vi "Write passerId.vi"(8 "error in (no error)":errorcluster, 10 "passerId":u8, 11 "PositionTactic in":refnum<class "PositionTactic.lvclass">) -> (0 "error out":errorcluster, 3 "PositionTactic out":refnum<class "PositionTactic.lvclass">)   [LabVIEW 2023, in "PositionTactic.lvclass"]
uses:
  PositionTactic.lvclass
  PositionTactic.lvclass/PositionTactic.ctl
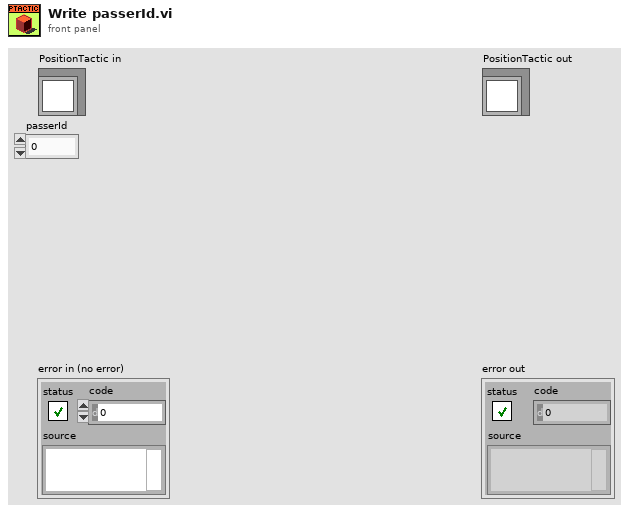
[diagram p1: front panel]
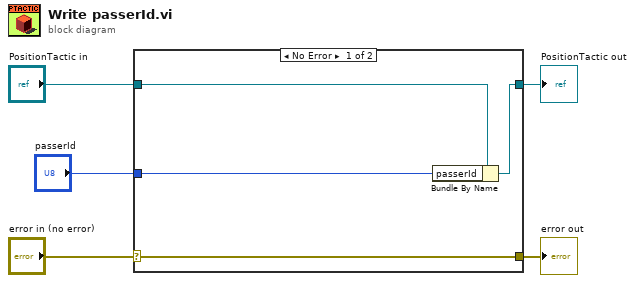
[diagram p0: block diagram]
diagram:
  n1 = case shown="No Error" "error in (no error)" {
    selector: "error in (no error)" -> [w9 w10]
    tunnel: [w9 w10] -> w4
    tunnel: [w7 w11] -> w2
    tunnel: "PositionTactic in" -> [w8 w11]
    tunnel: "passerId" -> [w6 _]
    frame No Error {
      n2 = Bundle By Name(cluster=w8, "passerId"=w6) -> (w7:refnum<class "PositionTactic.lvclass">)
    }
    frame Error {
    }
  }
  "error out" <- w4
  "PositionTactic out" <- w2
